vi "Get File Properties List.vi"(8 "error in (no error)":errorcluster, 11 "File Ref in":T1=18446744073709551615 format="%.0x") -> (0 "error out":errorcluster, 1 "System dt":dbl, 2 "Properties List":T2[](array[typedef]), 3 "File Ref out":T1=18446744073709551615 format="%.0x")   [LabVIEW 2027, in "Embedded Data Logger Engine.lvlib"]
uses:
  Embedded Data Logger Engine.lvlib
  Property Specification.ctl
  <vilib>/NI VeriStand/Custom Device API/Custom Device Item Ref.ctl
  <vilib>/NI VeriStand/Custom Device Tools/Custom Device Utility Library/Custom Device Utility Library.lvlib
  <vilib>/NI VeriStand/Custom Device API/Custom Device API.lvlib
  Scripting/Embedded Data Logger Scripting.lvlib
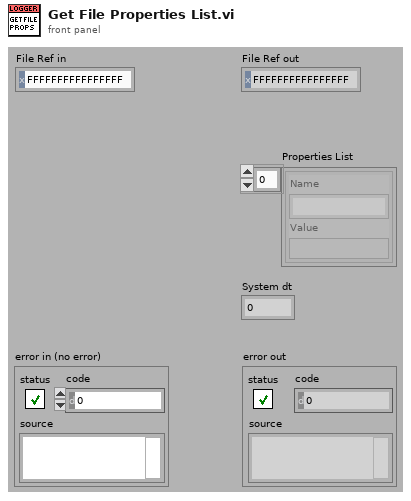
[diagram p1: front panel]
types:
  T1 = typedef "Custom Device API.lvlib/Custom Device Item Ref.ctl" = u64
  T2 = typedef "Embedded Data Logger Engine.lvlib/Property Specification.ctl" = cluster{"Name":string, "Value":variant}
  T3 = typedef "Custom Device API.lvlib/Custom Device Item Info.ctl" = cluster{"Name":string, "Is Channel":bool, "GUID":string, "Is Waveform":bool}
  T4 = typedef "Custom Device API.lvlib/Custom Device Channel.ctl" = cluster{"Type":T5, "Units":string, "Default Value":dbl, "Faultable":bool, "Scalable":bool}
  T5 = typedef "Custom Device API.lvlib/Custom Device Channel Type.ctl" = enum16{"Input", "Output"}
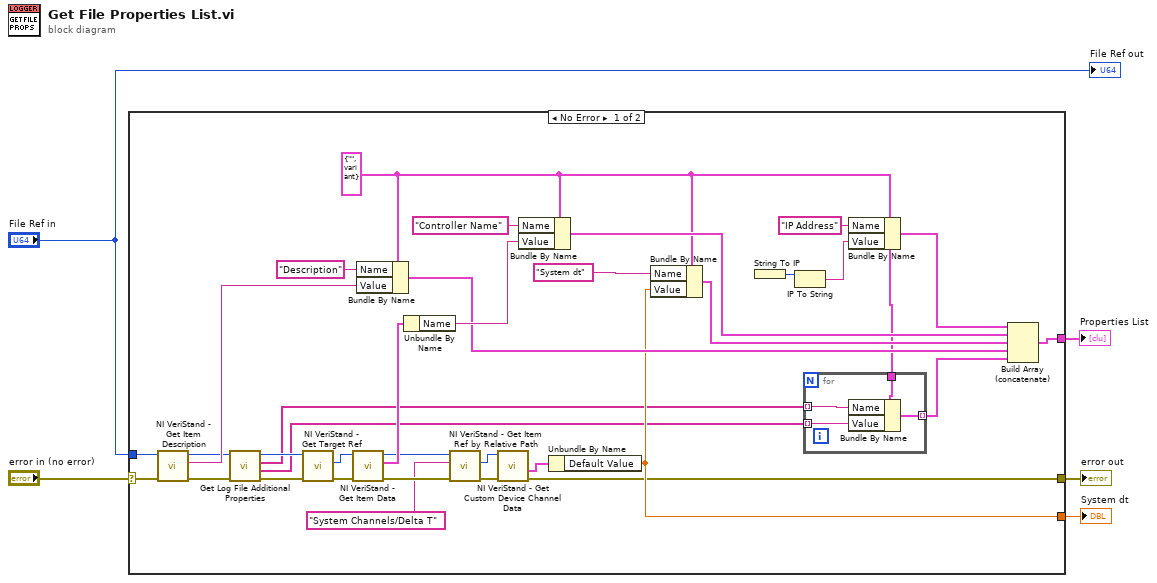
[diagram p0: block diagram]
diagram:
  n1 = case shown="No Error" "error in (no error)" {
    selector: "error in (no error)" -> [w20 w44]
    tunnel: [w14 w44] -> w5
    tunnel: [w39 _] -> w3
    tunnel: "File Ref in" -> [w21 _]
    tunnel: [w15 _] -> w1
    frame No Error {
      w6 = T2 {"Name"="", "Value"=variant} ("Property Spec")
      n2 = call <vilib>:"NI VeriStand - Get Item Description.vi"("error in (no error)"=w20, "Item Ref in"=w21) -> ("error out"=w19:errorcluster, "Description"=w17:string, "Item Ref out"=w11:T1)  [unwired: 7 out]
      n3 = call "Get Log File Additional Properties.vi"("error in"=w19, "log file in"=w11) -> ("error out"=w13:errorcluster, "property values"=w9:string[], "property names"=w10:string[], "log file out"=w12:T1)  [unwired: 6 in]
      n4 = call <vilib>:"NI VeriStand - Get Target Ref.vi"("error in"=w13, "Item Ref in"=w12) -> ("error out"=w32:errorcluster, "Target Ref"=w33:T1)  [unwired: 8 out]
      n5 = call <vilib>:"NI VeriStand - Get Item Data.vi"("error in (no error)"=w32, "Item Ref in"=w33) -> ("error out"=w28:errorcluster, "Item Info"=w31:T3, "Item Ref out"=w29:T1)  [unwired: 7 out]
      n6 = Bundle By Name(cluster=w6, "Name"="Description", "Value"=w17) -> (w16:T2)
      n7 = Unbundle By Name(w31) -> ("Name"=w30:string)
      n8 = call <vilib>:"NI VeriStand - Get Item Ref by Relative Path.vi"("error in"=w28, "Relative Item Path"="System Channels/Delta T", "Section Ref in"=w29) -> ("error out"=w25:errorcluster, "Item Ref"=w26:T1)  [unwired: 7 out]
      n9 = call <vilib>:"NI VeriStand - Get Custom Device Channel Data.vi"("error in (no error)"=w25, "Channel Ref in"=w26) -> ("error out"=w14:errorcluster, "Channel"=w24:T4)  [unwired: 8 out]
      n10 = Bundle By Name(cluster=w6, "Name"="Controller Name", "Value"=w30) -> (w34:T2)
      n11 = Unbundle By Name(w24) -> ("Default Value"=w15:dbl)
      n12 = Bundle By Name(cluster=w6, "Name"="System dt", "Value"=w15) -> (w22:T2)
      n13 = String To IP() -> (0:w37:u32)  [unwired: 1 out]
      n14 = IP To String(2:w37) -> (0:w36:string)  [unwired: 1 out]
      n15 = for {
        tunnel: w10 -> [w43] mode=indexing
        tunnel: w9 -> [w42] mode=indexing
        tunnel: [w41] -> w8 mode=indexing
        tunnel: w6 -> [w40]
        n16 = Bundle By Name(cluster=w40, "Name"=w43, "Value"=w42) -> (w41:T2)
      }
      n17 = Bundle By Name(cluster=w6, "Name"="IP Address", "Value"=w36) -> (w7:T2)
      n18 = Build Array (concatenate)(w7, w34, w22, w16, w8) -> (w39:T2[])
    }
    frame Error {
    }
  }
  "error out" <- w5
  "Properties List" <- w3
  "System dt" <- w1
  "File Ref out" <- "File Ref in"
